vi "Table_Sort.vi"(7 "Sort Type":enum16{"numerical", "string"}(ring), 9 "Sort by":u16(ring) items=["Packet_Number", "Timestamp", "Source", "Destination", "Protocol", "Length", "Data"], 11 "Unsorted Data":string[][](array[string])=array1500x7[10500 elements]) -> (3 "Sorted data":string[][](array[string]))   [LabVIEW 2025, in "Table_Filtering.lvlib"]
uses:
  Table_Filtering.lvlib
  dd903b07-9a56-4d29-89d8-b4a603456dcb.vi
  <vilib>/Array/Sort 2D Array - Pop Stack.vi
  <vilib>/Array/Sort 2D Array - Push Stack.vi
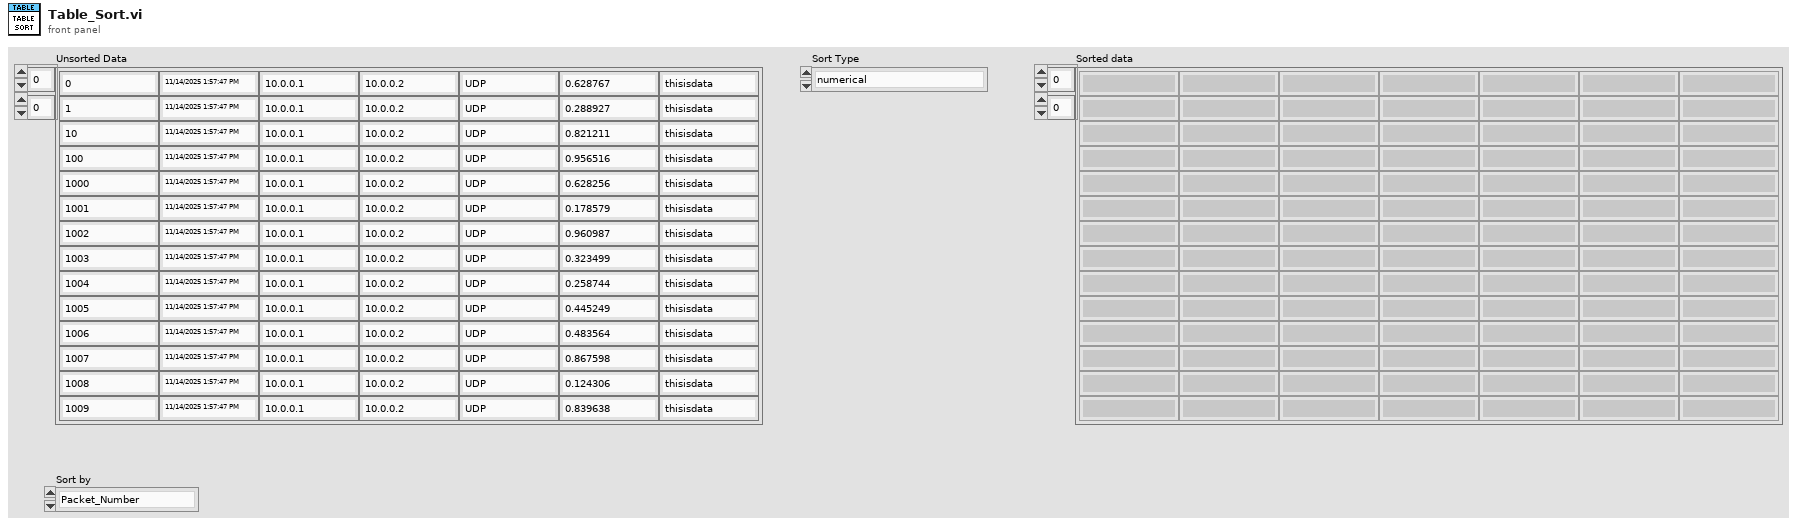
[diagram p1: front panel]
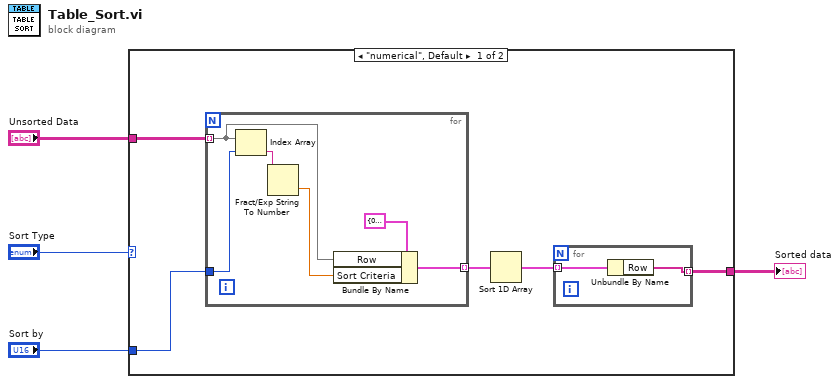
[diagram p0: block diagram]
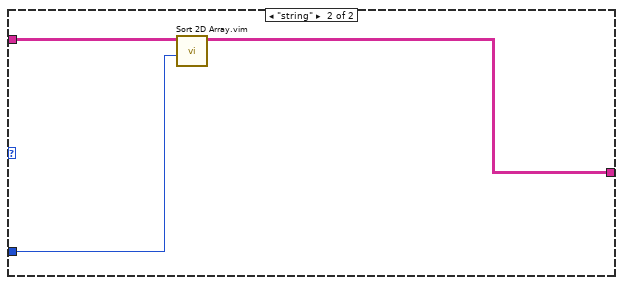
[diagram p2: hidden frame]
diagram:
  n1 = case shown="\"numerical\", Default" "Sort Type" {
    tunnel: "Unsorted Data" -> [w9 w20]
    tunnel: "Sort by" -> [w8 w18]
    tunnel: [w5 w19] -> w1
    frame "numerical", Default {
      n2 = for {
        tunnel: w9 -> [w14] mode=indexing
        tunnel: w8 -> [w15]
        tunnel: [w12] -> w7 mode=indexing
        n3 = Index Array(array=w14, index=w15) -> (element=w17:string)
        n4 = Fract/Exp String To Number(string=w17) -> (number=w13:dbl)  [unwired: 3 in, 1 out]
        n5 = Bundle By Name(cluster=cluster{"Sort Criteria":dbl, "Row":string[]} {"Sort Criteria"=0.0, "Row"=[]}, "Row"=w14, "Sort Criteria"=w13) -> (w12:cluster{"Sort Criteria":dbl, "Row":string[]})
      }
      n6 = Sort 1D Array(array=w7) -> (sorted array=w6:cluster{"Sort Criteria":dbl, "Row":string[]}[])
      n7 = for {
        tunnel: w6 -> [w11] mode=indexing
        tunnel: [w10] -> w5 mode=indexing
        n8 = Unbundle By Name(w11) -> ("Row"=w10:string[])
      }
    }
    frame "string" {
      n9 = call "Sort 2D Array.vim"("index"=w18, "2D array"=w20) -> ("sorted 2D array"=w19:string[][])  [unwired: 8 in, 1 out]
    }
  }
  "Sorted data" <- w1
